vi "Set Edge Trigger.vi"(6 "Trigger Slope (0: Rising)":u16(ring) items=["Rising", "Falling", "Either"], 7 "Trigger Coupling (0 : DC)":u16(ring) items=["DC", "HF Reject", "LF Reject", "Noise Reject", "AC"], 8 "error in (no error)":errorcluster, 9 "Trigger Level (0.0 V)":dbl, 10 "Analog Channel":T1, 11 "MSOX6004 in":refnum<class "MSOX6004.lvclass">) -> (0 "error out":errorcluster, 3 "MSOX6004 out":refnum<class "MSOX6004.lvclass">)   [LabVIEW 2018, in "MSOX6004.lvlib" / "MSOX6004.lvclass"]
uses:
  MSOX6004.lvclass
  PPLs/Oscilloscope/Parent/Oscilloscope.lvlibp/Custom Controls/Analog Channels.ctl
  MSOX6004.lvclass/MSOX6004.ctl
  <instrlib>/Keysight InfiniiVision/Keysight InfiniiVision.lvlib
  PPLs/Oscilloscope/Parent/Oscilloscope.lvlibp
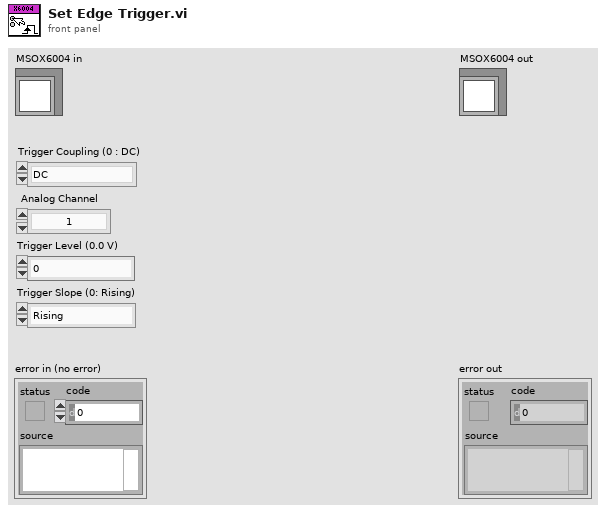
[diagram p1: front panel]
types:
  T1 = typedef "Oscilloscope.lvlibp/Analog Channels.ctl" = enum16{"1", "2", "3", "4", "5", "6", "7", "8", "9", "10", "11", "12", "13", "14", "15", "16"}
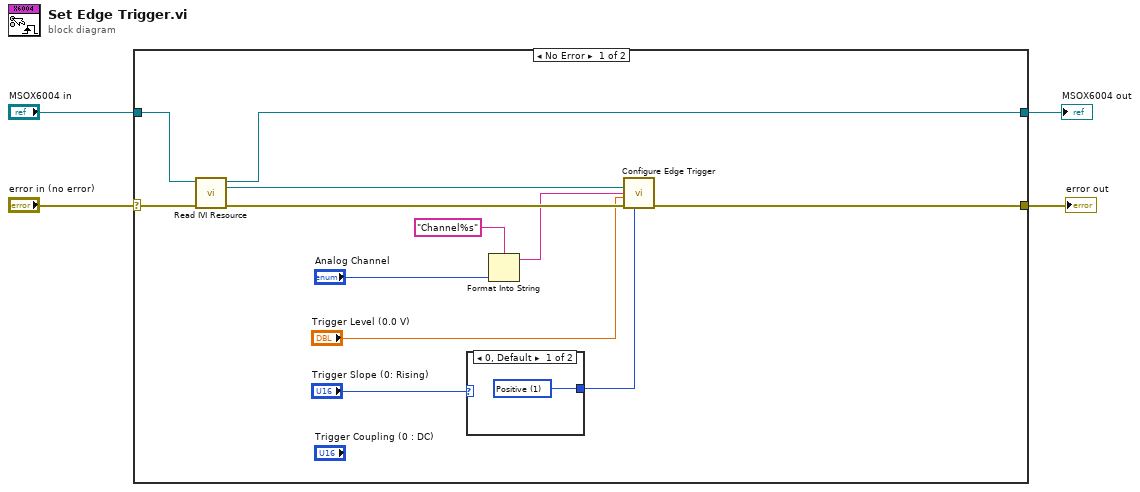
[diagram p0: block diagram]
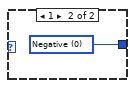
[diagram p2: hidden frame]
diagram:
  n1 = case shown="No Error" "error in (no error)" {
    selector: "error in (no error)" -> [w16 w20]
    tunnel: [w5 w20] -> w3
    tunnel: [w14 w19] -> w2
    tunnel: "MSOX6004 in" -> [w15 w19]
    frame No Error {
      n2 = call "Read IVI Resource.vi"("error in (no error)"=w16, "MSOX6004 in"=w15) -> ("error out"=w13:errorcluster, "IVI Resource"=w12:refnum<k15>, "MSOX6004 out"=w14:refnum<class "MSOX6004.lvclass">)  [unwired: 7 in]
      n3 = case shown="0, Default" "Trigger Slope (0: Rising)" {
        tunnel: [w17 w18] -> w10
        frame 0, Default {
          w17 = 1 items=["Negative", "Positive"] ("trigger slope (Negative)")
        }
        frame 1 {
          w18 = 0 items=["Negative", "Positive"] ("trigger slope (Negative)")
        }
      }
      n4 = Format Into String(format string="Channel%s", "Analog Channel") -> (resulting string=w6:string)  [unwired: 2 in, 1 out]
      n5 = call <instrlib>:"Configure Edge Trigger.vi"("trigger slope (Negative)"=w10, "error in (no error)"=w13, "trigger level"="Trigger Level (0.0 V)", "trigger source"=w6, "instrument handle"=w12) -> ("error out"=w5:errorcluster)  [unwired: 5 in, 1 out]
    }
    frame Error {
    }
  }
  "error out" <- w3
  "MSOX6004 out" <- w2
